vi "Queue_Alarmas.vi"() -> ()   [LabVIEW 2018]
panel:
  in  "queue_alarma":refnum<queue>
  in  "queue_alarmas_G06":refnum<queue>
  in  "queue_alarmas_G05":refnum<queue>
  in  "queue_alarmas_G04":refnum<queue>
  in  "queue_alarmas_G03":refnum<queue>
  in  "queue_alarmas_G02":refnum<queue>
  in  "queue_alarmas_G01":refnum<queue>
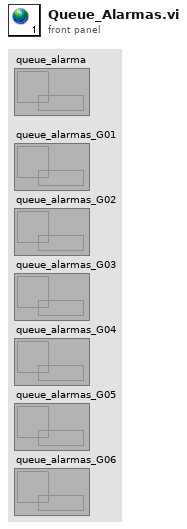
[diagram p1: front panel]
diagram:
